vi "ADAM 5000 Get Temperatures.vi"(11 "Remote IP Address 2":string="192.168.10.200") -> (1 "TC String Array":string[](array[string])=["347.07", "346.79", "346.79", "347.07", "347.34", "347.07", "347.34", "1369.68", "1369.68", "1369.68", "1369.68", "1369.68", "1369.68", "1369.68"], 2 "TC Array":dbl[](array[numeric])=[347.06539999999995, 346.7937, 346.7937, 347.06539999999995, 347.33709999999996, 347.06539999999995, 347.33709999999996, 1369.6815, 1369.6815, 1369.6815, 1369.6815, 1369.6815, 1369.6815])   [LabVIEW 2018]
uses:
  Adam Stuff/nimodbus121/71/vi.lib/NI Modbus.llb/MB Modbus Command.ctl
panel:
  out "error out":errorcluster
  in  "Modbus Command":T1={"Function Code"=3, "Starting Address"=48, "Quantity"=15, "Data"=[], "Discrete"=[]} {"Function Code" items=["Read Coils"=1, "Read Discrete Inputs"=2, "Read Holding Registers"=3, "Read Input Registers"=4, "Write Single Coil"=5, "Write Single Register"=6, "Read Exception Status"=7, "Write Multiple Coils"=15, "Write Multiple Registers"=16]}
  out "Slave Input Registers 1":u16[](array[numeric])=[16606, 16593, 16593, 16606, 16619, 16606, 16619, 0, 65535, 65535, 65535, 65535, 65535, 65535, 65535] caption="Slave Input Registers (Read Only)"
  in  "Remote Port 2":u16=502
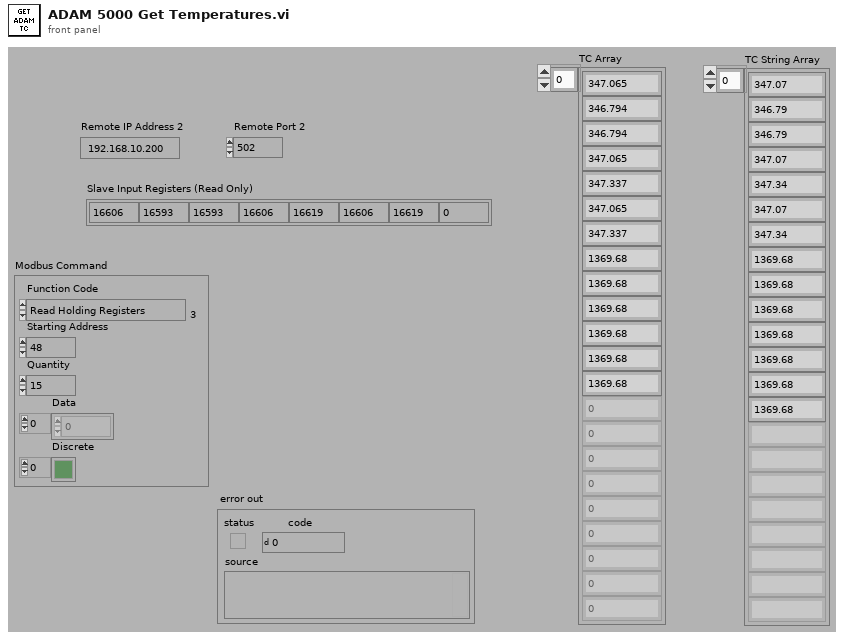
[diagram p1: front panel]
types:
  T1 = typedef "MB Modbus Command.ctl" = cluster{"Function Code":u8, "Starting Address":u16, "Quantity":u16, "Data":u16[], "Discrete":bool[]}
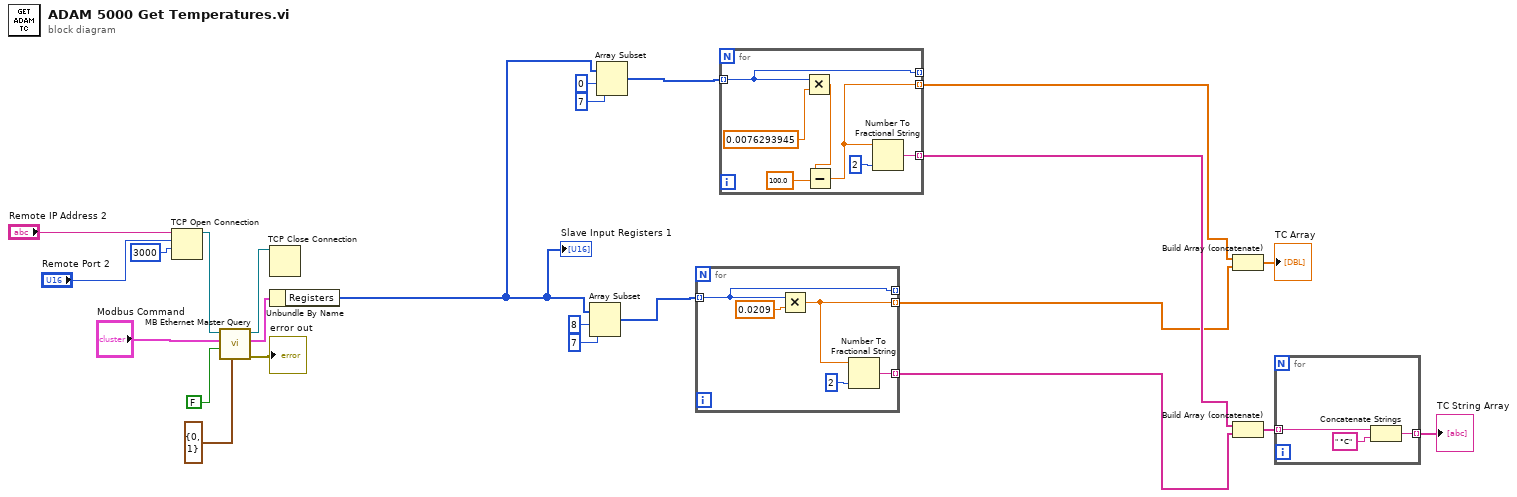
[diagram p0: block diagram]
diagram:
  n1 = TCP Open Connection(address="Remote IP Address 2", remote port or service name="Remote Port 2", timeout ms (60000)=3000) -> (connection ID=w22:refnum<k5>)  [unwired: 2 in, 1 out]
  n2 = call "MB Ethernet Master Query.vi"("MBAP Header"=cluster{"Transaction ID":u16, "Unit ID":u8} {"Transaction ID"=0, "Unit ID"=1}, "Use MODBUS Data Unit?"=FALSE, "Modbus Command"="Modbus Command", "TCP Connection Refnum in"=w22) -> ("error out"=→"error out":errorcluster, "Registers"=w18:cluster{"Registers":u16[], "Discrete":bool[]}, "TCP Connection Refnum (dup)"=w21:refnum<k5>)  [unwired: 3 in, 2 out]
  n3 = TCP Close Connection(connection ID=w21) -> ()  [unwired: 2 in, 2 out]
  n4 = Unbundle By Name(w18) -> ("Registers"=w6:u16[])
  "Slave Input Registers 1" <- w6
  n5 = Array Subset(array=w6, index=8, length=7) -> (w9:u16[])
  n6 = Array Subset(array=w6, index=0, length=7) -> (w5:u16[])
  n7 = for {
    tunnel: w9 -> [w25] mode=indexing
    tunnel: [w28] -> w1 mode=indexing
    tunnel: [w26] -> w3 mode=indexing
    tunnel: [w25] -> _ mode=indexing
    n8 = Multiply(x=w25, y=0.0209) -> (x*y=w28:dbl)
    n9 = Number To Fractional String(number=w28, precision (6)=i16 2) -> (F-format string=w26:string)  [unwired: 2 in]
  }
  n10 = for {
    tunnel: w5 -> [w33] mode=indexing
    tunnel: [w30] -> w2 mode=indexing
    tunnel: [w34] -> w4 mode=indexing
    tunnel: [w33] -> _ mode=indexing
    n11 = Multiply(x=w33, y=0.0076293945) -> (x*y=w32:dbl)
    n12 = Subtract(x=w32, y=100.0) -> (x-y=w30:dbl)
    n13 = Number To Fractional String(number=w30, precision (6)=i16 2) -> (F-format string=w34:string)  [unwired: 2 in]
  }
  n14 = Build Array (concatenate)(w2, w1) -> (→"TC Array":dbl[])
  n15 = Build Array (concatenate)(w4, w3) -> (w13:string[])
  n16 = for {
    tunnel: w13 -> [w39] mode=indexing
    tunnel: [w37] -> w12 mode=indexing
    n17 = Concatenate Strings(w39, " °C") -> (w37:string)
  }
  "TC String Array" <- w12
